vi "ValidateWSDL.vi"(8 "error in (no error)":errorcluster, 9 "Proxy Server Info":T1, 10 "Web Service Authentication":T2, 11 "URL in":string) -> (0 "error out":errorcluster, 2 "ErrorCode":i32(ring)=200 items=["kNoError"=200, "kUnknownError"=201, "kBadArgument"=202, "kUrlNotFoundOrBadWSDL"=203, "kBadlyFormattedURL"=204, "kBadHostname"=205], 3 "Web Service Importer Ref":refnum<k24>)   [LabVIEW 2020]
uses:
  e:/builds/penguin/labview/branches/2020/dev/dist/resource/WebServiceUtils.dll
  resource/WebServiceUtils.dll
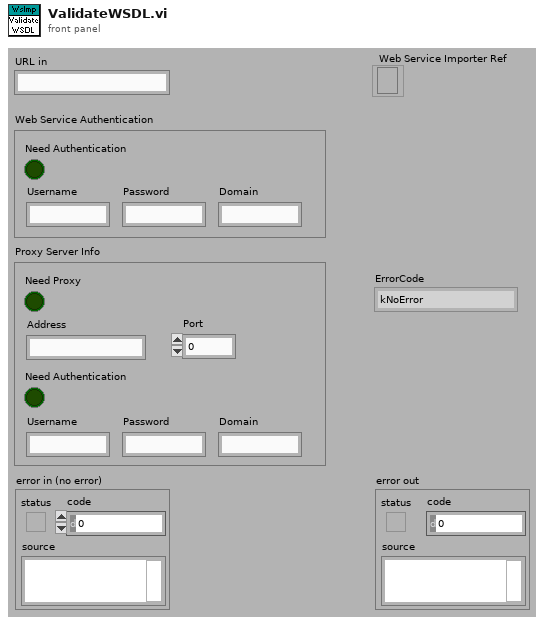
[diagram p1: front panel]
types:
  T1 = cluster{"Need Proxy":bool, "Username":string, "Password":string, "Domain":string, "Address":string, "Port":i32, "Need Authentication":bool}
  T2 = cluster{"Need Authentication":bool, "Username":string, "Password":string, "Domain":string}
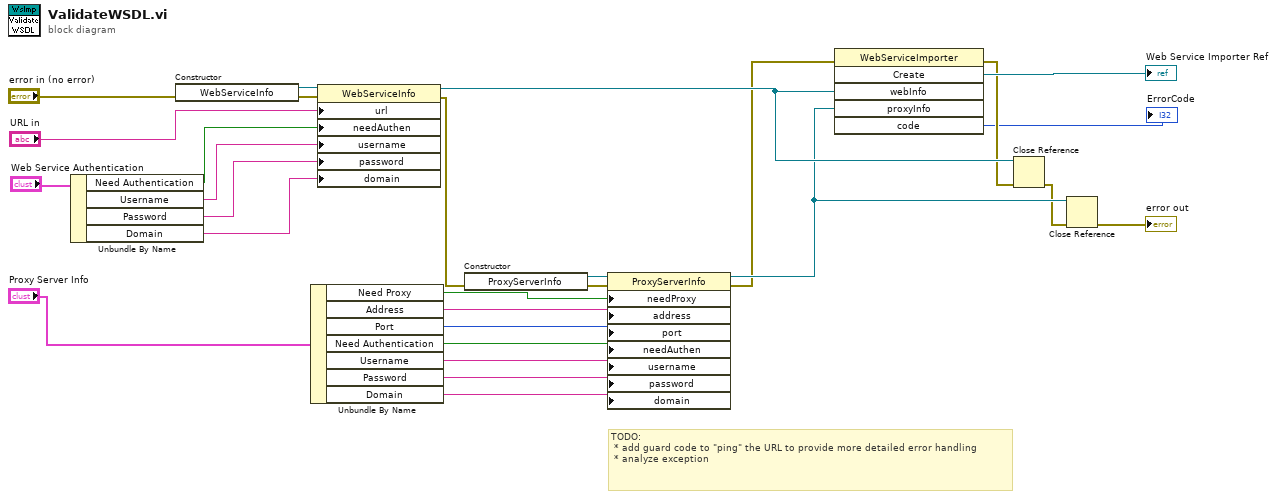
[diagram p0: block diagram]
diagram:
  # "TODO: \n * add guard code to \"ping\" the URL to provide more detailed error handling\n * analyze exception"
  n1 = Unbundle By Name("Web Service Authentication") -> ("Need Authentication"=w22:bool, "Username"=w21:string, "Password"=w20:string, "Domain"=w19:string)
  n2 = constructor class="WebServiceInfo"(error in="error in (no error)") -> (reference out=w27:refnum<k24>, error out=w26:errorcluster)  [unwired: 2 in, 1 out]
  n3 = Unbundle By Name("Proxy Server Info") -> ("Need Proxy"=w8:bool, "Address"=w7:string, "Port"=w1:i32, "Need Authentication"=w6:bool, "Username"=w5:string, "Password"=w4:string, "Domain"=w3:string)
  n4 = property class="WebServiceInfo"(reference=w27, error in=w26, "url"="URL in", "needAuthen"=w22, "username"=w21, "password"=w20, "domain"=w19) -> (reference out=w16:refnum<k24>, error out=w10:errorcluster)
  n5 = constructor class="ProxyServerInfo"(error in=w10) -> (reference out=w2:refnum<k24>, error out=w18:errorcluster)  [unwired: 2 in, 1 out]
  n6 = property class="ProxyServerInfo"(reference=w2, error in=w18, "needProxy"=w8, "address"=w7, "port"=w1, "needAuthen"=w6, "username"=w5, "password"=w4, "domain"=w3) -> (reference out=w14:refnum<k24>, error out=w9:errorcluster)
  n7 = invoke class="WebServiceImporter" method="Create"(error in=w9, "webInfo"=w16, "proxyInfo"=w14) -> (error out=w15:errorcluster, "Create"=→"Web Service Importer Ref":refnum<k24>, "code"=→"ErrorCode":i32)  [unwired: 3 in, 3 out]
  n8 = Close Reference(reference=w16, error in (no error)=w15) -> (error out=w13:errorcluster)
  n9 = Close Reference(reference=w14, error in (no error)=w13) -> (error out=→"error out":errorcluster)
